vi "Configure AO.vi"(8 "error in (no error)":errorcluster, 10 "AO Channels":tag, 11 "DAQ HVPS in":refnum<class "DAQ HVPS.lvclass">) -> (0 "error out":errorcluster, 3 "DAQ HVPS out":refnum<class "DAQ HVPS.lvclass">)   [LabVIEW 2014, in "DAQ HVPS.lvclass"]
uses:
  DAQ HVPS.lvclass
  DAQ HVPS.lvclass/DAQ HVPS.ctl
  <vilib>/DAQmx/create/scale.llb/DAQmx Create Scale (Linear).vi
  <vilib>/DAQmx/create/channels.llb/DAQmx Create Channel (AO-Voltage-Basic).vi
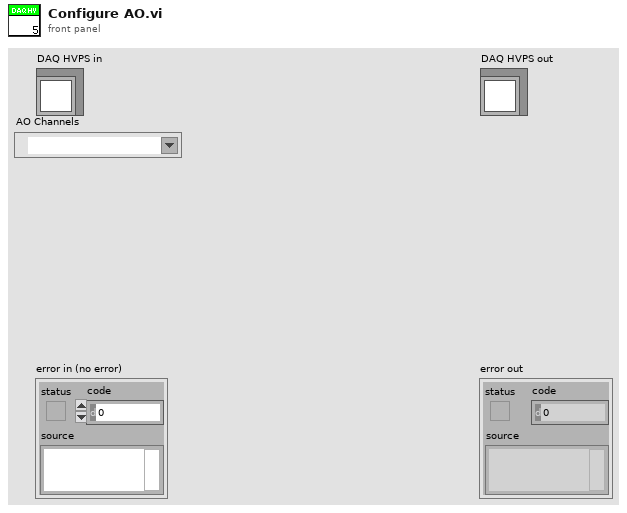
[diagram p1: front panel]
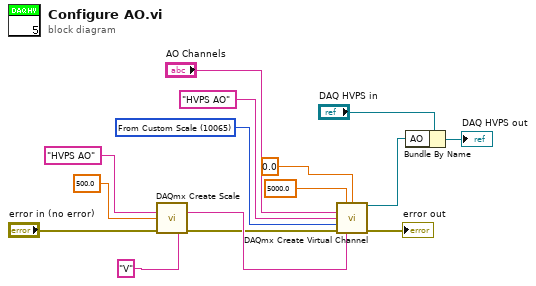
[diagram p0: block diagram]
diagram:
  w14 = 10065 items=["Volts"=10348, "From Custom Scale"=10065] ("units")
  n1 = call-poly <vilib>:"DAQmx Create Scale.vi"("name"="HVPS AO", "slope"=500.0, "error in"="error in (no error)", "scaled units"="V") -> ("scale out"=w10:tag, "error out"=w9:errorcluster)  [unwired: 10 in]
  n2 = call-poly <vilib>:"DAQmx Create Virtual Channel.vi"("maximum value"=5000.0, "minimum value"=0.0, "physical channels"="AO Channels", "name to assign"="HVPS AO", "units"=w14, "error in"=w9, "custom scale name"=w10) -> ("task out"=w4:refnum<k21>, "error out"=→"error out":errorcluster)  [unwired: 7 in]
  n3 = Bundle By Name(cluster="DAQ HVPS in", "AO"=w4) -> (→"DAQ HVPS out":refnum<class "DAQ HVPS.lvclass">)
